vi "NI Vision Get ROIs.vi"() -> ()   [LabVIEW 2015]
panel:
  out "ROI":T1
  out "Image":T2(plugin-control)
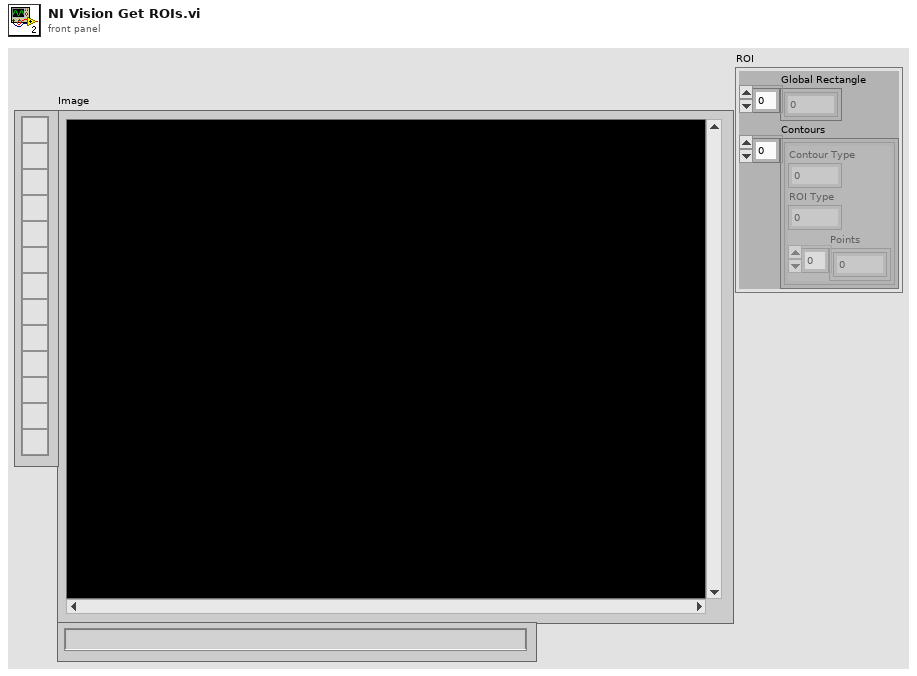
[diagram p1: front panel]
types:
  T1 = cluster{"Global Rectangle":i32[], "Contours":cluster{"Contour Type":u32, "ROI Type":u32, "Points":i32[]}[]}
  T2 = typedef "IMAQ Image.ctl" = refnum<image>
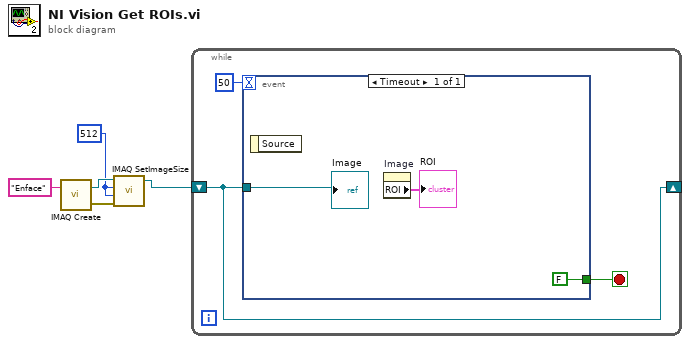
[diagram p0: block diagram]
diagram:
  w1 = 512 ("X Resolution")
  n1 = call "IMAQ Create"("Image Name"="Enface") -> ("New Image"=w3:T2, "error out"=w4:errorcluster)  [unwired: 4 in]
  n2 = call "IMAQ SetImageSize"("error in (no error)"=w4, "Y Resolution"=w1, "X Resolution"=w1, "Image"=w3) -> ("Image Out"=w2:T2)  [unwired: 1 in, 1 out]
  n3 = while {
    shift-right: [w6] -> _
    shift-left: w2 -> [w6]
    stop <- w8 stop-if-true
    n4 = event shown="[0] Timeout" {
      selector: _ -> [_]
      dyn-events: _ -> [_]
      timeout: 50 -> [_]
      tunnel: [FALSE] -> w8
      tunnel: w6 -> [w9]
      event Timeout {
        n5 = event-data() -> ()  [unwired: 1 in, 1 out]
        n6 = property on="Image" class="ImageControl"() -> ("ROI"=→"ROI":T1)  [unwired: 2 in, 2 out]
        "Image" <- w9
      }
    }
  }
